vi "KundtsTube.vi"() -> ()   [LabVIEW 2014]
doc: "This VI measures response from a Kundt's tube. The VI sends a signal to a speaker in the tube and then measures the response. The user can sweep through a range of frequencies or input a single frequency. The VI plots the data of the sweep and also saves it as a spreadsheet text file."
uses:
  <vilib>/Utility/file.llb/Write To Spreadsheet File (DBL).vi
panel:
  out "Frequency":dbl=10000.0
  out "RMS Voltage":dbl=0.011041164052449856 format="%0.2f"
  out "Gain vs. Sweep Frequency":cluster{dbl[], dbl[]}(graph)
  out "Oscilliscope":dynamicdata(graph)=[{"t0"=timestamp(3497985160.405834 s since 1904-01-01), "dt"=9.999999999999972e-06, "Y"=array[1000 elements], "attributes"=variant("NI_ChannelName"=variant(string "Voltage"), "NI_UnitDescription"=variant(string "Volts"))}]
  in  "Rate":dbl=100000.0
  in  "Number of Samples":i32=1000
  out "error out":errorcluster
  in  "stop":bool
  in  "Amplitude":dbl=2.0
  in  "Sweep Parameters":T1={"Minimum"=10.0, "Maximum"=10000.0, "# of Points"=500.0, "Spacing"=enum."Linear"}
  in  "Type of Measurement":enum32{"Sweep", "Single"}(tab)
  in  "Dwell Time (s)":dbl=1.0
  in  "Single Frequency":dbl=504.0
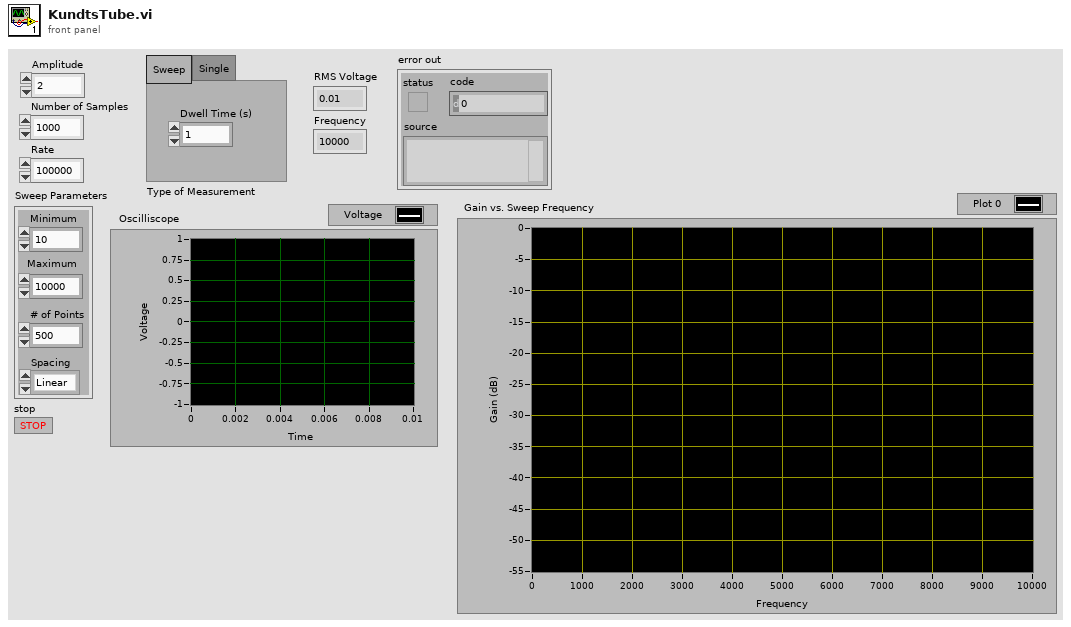
[diagram p1: front panel]
types:
  T1 = cluster{"Minimum":dbl, "Maximum":dbl, "# of Points":dbl, "Spacing":enum16{"Linear", "Logarithmic"}}
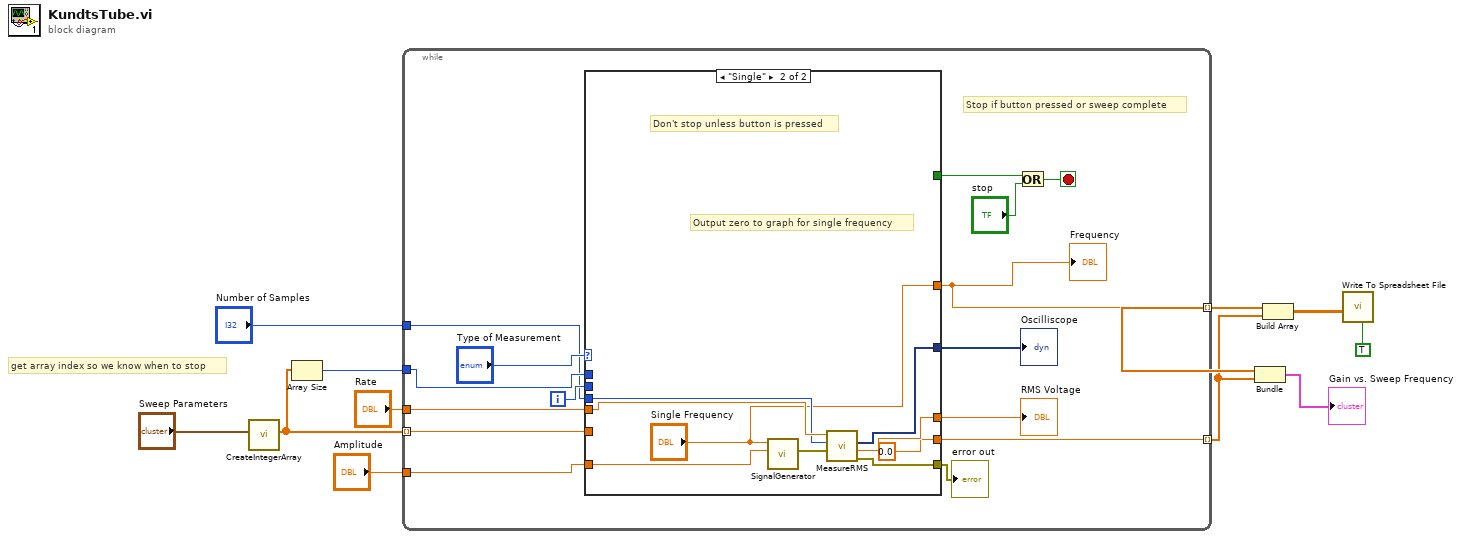
[diagram p0: block diagram]
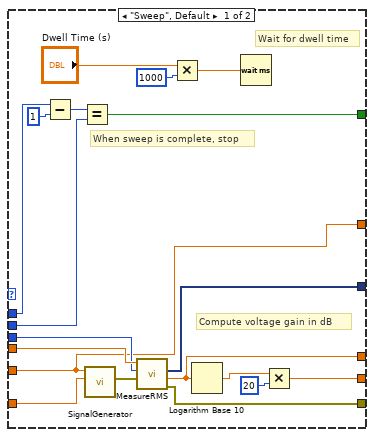
[diagram p2: hidden frame]
diagram:
  # "get array index so we know when to stop"
  n1 = call "CreateIntegerArray.vi"("Cluster"="Sweep Parameters") -> ("Output Array"=w8:dbl[])  [unwired: 10 in]
  n2 = Array Size(array=w8) -> (size(s)=w7:i32)
  n3 = while {
    tunnel: w8 -> [w25] mode=indexing
    tunnel: "Amplitude" -> [w24]
    tunnel: [w12] -> w4 mode=indexing
    tunnel: [w14] -> w3 mode=indexing
    tunnel: w7 -> [w23]
    tunnel: "Rate" -> [w16]
    tunnel: "Number of Samples" -> [w15]
    i -> [w22]
    stop <- w19 stop-if-true
    # "Stop if button pressed or sweep complete"
    n4 = case shown="\"Single\"" "Type of Measurement" {
      tunnel: w25 -> [w32 _]
      tunnel: w24 -> [w45 w54]
      tunnel: w23 -> [w39 _]
      tunnel: w22 -> [w41 _]
      tunnel: [w40 _] -> w20
      tunnel: [w33 w52] -> w18
      tunnel: [w28 w51] -> w17
      tunnel: w16 -> [w35 w50]
      tunnel: w15 -> [w34 w49]
      tunnel: [w29 0.0] -> w14
      tunnel: [w32 "Single Frequency"] -> w12
      tunnel: [w27 w46] -> w13
      frame "Sweep", Default {
        # "Compute voltage gain in dB"
        # "Wait for dwell time"
        # "When sweep is complete, stop"
        n5 = Subtract(x=w39, y=1) -> (x-y=w37:i32)
        n6 = Equal?(x=w37, y=w41) -> (x = y?=w40:bool)
        n7 = call "SignalGenerator.vi"("Amplitude"=w45, "Frequency"=w32) -> ("error out"=w36:errorcluster)  [unwired: 9 in]
        n8 = call "MeasureRMS.vi"("error in"=w36, "Number of Samples"=w34, "Rate"=w35) -> ("error out"=w33:errorcluster, "RMS Voltage"=w28:dbl, "Waveform Graph"=w27:dynamicdata)  [unwired: 6 in]
        n9 = Multiply(x="Dwell Time (s)", y=1000) -> (x*y=w43:dbl)
        n10 = Logarithm Base 10(1:w28) -> (0:w31:dbl)
        n11 = Wait (ms)(milliseconds to wait=w43) -> ()  [unwired: 1 out]
        n12 = Multiply(x=w31, y=20) -> (x*y=w29:dbl)
      }
      frame "Single" {
        # "Don't stop unless button is pressed"
        # "Output zero to graph for single frequency"
        n13 = call "SignalGenerator.vi"("Amplitude"=w54, "Frequency"="Single Frequency") -> ("error out"=w53:errorcluster)  [unwired: 9 in]
        n14 = call "MeasureRMS.vi"("error in"=w53, "Number of Samples"=w49, "Rate"=w50) -> ("error out"=w52:errorcluster, "RMS Voltage"=w51:dbl, "Waveform Graph"=w46:dynamicdata)  [unwired: 6 in]
      }
    }
    "error out" <- w18
    "RMS Voltage" <- w17
    "Frequency" <- w12
    "Oscilliscope" <- w13
    n15 = Or(x=w20, y="stop") -> (x .or. y?=w19:bool)
  }
  n16 = Bundle(w4, w3) -> (→"Gain vs. Sweep Frequency":cluster{dbl[], dbl[]})  [unwired: 1 in]
  n17 = Build Array(w4, w3) -> (w2:dbl[][])
  n18 = call-poly <vilib>:"Write To Spreadsheet File.vi"("transpose? (no:F)"=TRUE, "2D data"=w2) -> ()  [unwired: 6 in, 1 out]
